vi "appendText.vi"(8 "error in (no error)":errorcluster, 9 "Style":refnum<class "Style.lvclass">, 10 "Text":string, 11 "MS-Excel in":refnum<class "MS-Excel.lvclass">) -> (0 "error out":errorcluster, 3 "MS-Excel out":refnum<class "MS-Excel.lvclass">)   [LabVIEW 2017, in "LabVIEW NPOI.lvlib" / "MS-Excel.lvclass"]
uses:
  MS-Excel.lvclass
  Styles/Style/Style.lvclass
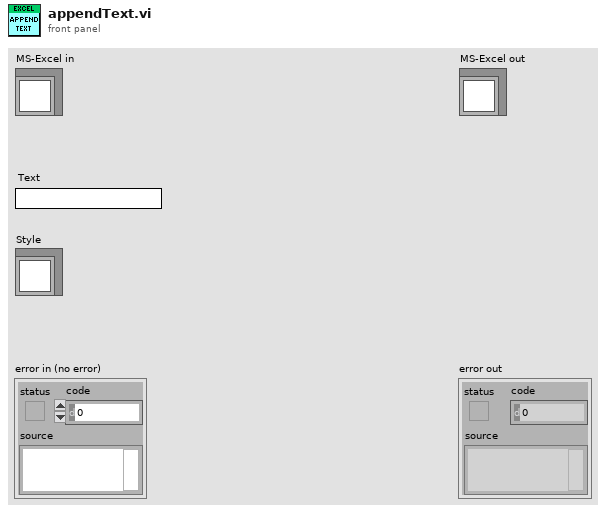
[diagram p1: front panel]
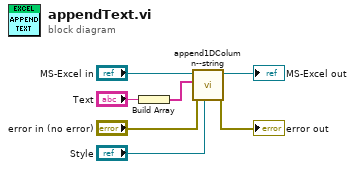
[diagram p0: block diagram]
diagram:
  n1 = Build Array("Text") -> (w5:string[])
  n2 = call-dynamic "append1DColumn--string.vi"("Style"="Style", "error in (no error)"="error in (no error)", "Value"=w5, "MS-Excel in"="MS-Excel in") -> ("error out"=→"error out":errorcluster, "MS-Excel out"=→"MS-Excel out":refnum<class "MS-Excel.lvclass">)  [unwired: 6 in]
